vi "Vision.vi"(7 "error in":errorcluster) -> (27 "error out":errorcluster)   [LabVIEW 2015]
uses:
  <vilib>/vision/NI_Vision_Development_Module.lvlib
panel:
  out "Image Out":T1(plugin-control)
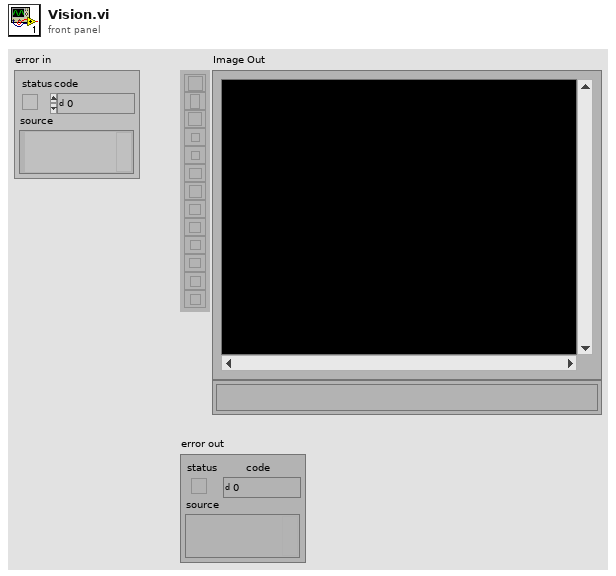
[diagram p1: front panel]
types:
  T1 = typedef "IMAQ Image.ctl" = refnum<image>
  T2 = typedef "Image Type" = u32
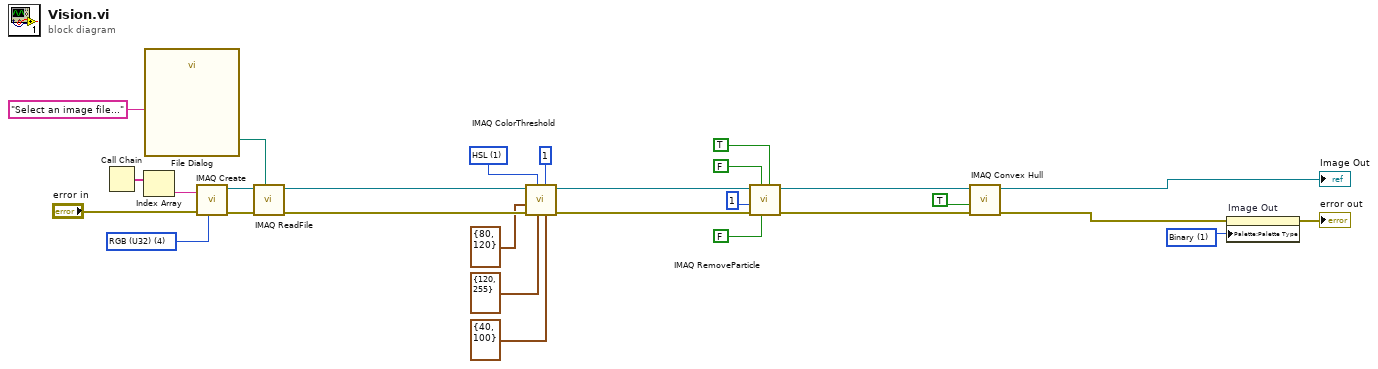
[diagram p0: block diagram]
diagram:
  w1 = u32 1 items=["Grayscale", "Binary", "Gradient", "Rainbow", "Temperature", "User Defined", "Binary 16 Bit", "Gradient 16 Bit", "Rainbow 16 Bit", "Temperature 16 Bit", "User Defined 16 Bit"] ("Palette Type")
  w18 = u16 1 items=["RGB", "HSL", "HSV", "HSI"] ("Color Mode")
  w20 = T2 4 items=["Grayscale (U8)", "Grayscale (I16)", "Grayscale (SGL)", "Complex (CSG)", "RGB (U32)", "HSL (U32)", "RGB (U64)", "Grayscale (U16)"] ("Image Type")
  n1 = Call Chain() -> (call chain=w24:string[])
  n2 = Index Array(array=w24) -> (element=w23:string)  [unwired: 1 in]
  n3 = call "File Dialog"("prompt"="Select an image file...") -> ("selected path"=w21:path)  [unwired: 6 in, 8 out]
  n4 = call "IMAQ Create"("Image Name"=w23, "Image Type"=w20, "error in (no error)"="error in") -> ("New Image"=w27:T1, "error out"=w26:errorcluster)  [unwired: 1 in, 1 out]
  n5 = call "IMAQ ReadFile"("File Path"=w21, "error in (no error)"=w26, "Image"=w27) -> ("error out"=w28:errorcluster, "Image Out"=w14:T1)  [unwired: 2 in, 5 out]
  n6 = call "IMAQ ColorThreshold"("Blue or Luma or Val or Inten Range"=cluster{"Lower value":i32, "Upper value":i32} {"Lower value"=40, "Upper value"=100}, "Replace Value"=1, "Green or Sat Range"=cluster{"Lower value":i32, "Upper value":i32} {"Lower value"=120, "Upper value"=255}, "Color Mode"=w18, "error in (no error)"=w28, "Red or Hue Range"=cluster{"Lower value":i32, "Upper value":i32} {"Lower value"=80, "Upper value"=120}, "Image Src"=w14) -> ("error out"=w13:errorcluster, "Image Dst Out"=w8:T1)  [unwired: 1 in, 2 out]
  n7 = call "IMAQ RemoveParticle"("Connectivity 4/8 (8)"=TRUE, "Low Pass/High Pass (Low)"=FALSE, "Square/Hexa (Square)"=FALSE, "error in (no error)"=w13, "Number of Erosion"=1, "Image Src"=w8) -> ("error out"=w7:errorcluster, "Image Dst Out"=w6:T1)  [unwired: 1 in, 3 out]
  n8 = call "IMAQ Convex Hull"("error in (no error)"=w7, "Connectivity 4/8 (8)"=TRUE, "Image Src"=w6) -> ("error out"=w4:errorcluster, "Image Dst Out"=→"Image Out":T1)  [unwired: 1 in, 6 out]
  n9 = property on="Image Out" class="ImageControl"(error in=w4, "Palette:Palette Type"=w1) -> (error out=→"error out":errorcluster)  [unwired: 1 in, 1 out]
